vi "SelfieStickControl.vi"(5 "Home Complete":bool, 6 "Arm Position":T23, 7 "Manual Control":dbl, 8 "Inhibit Extend":bool, 9 "Manual Toggle":bool, 10 "Selfie Stick Motor DevRef":T2={"DeviceStatus"={"status"=FALSE, "code"=0, "source"=""}, "Type"=enum."PWM", "PWM"={"PWM Channel"=enum."Invalid", "DeadBand"={"Name"="", "maxPositivePwm"=0, "minPositivePwm"=0, "centerPwm"=0, "maxNegativePwm"=0, "minNegativePwm"=0, "angularRange"=0}}, "CAN"={"Device Number"=0, "SetOutput VI Ref"=variant(enum8{"Percent VBus", "Current", "Speed", "Position", "Voltage"} enum."Percent VBus"), "GetOutput VI Ref"=variant(refnum<k1> refnum), "Enable VI Ref"=variant(dbl 12.0), "Disable VI Ref"=variant(enum8{"Percent VBus", "Speed", "Position", "Slave", "Unchanged / Invalid", "Voltage Compensation", "Current", "Motion Profile"} enum."Percent VBus"), "Data"=variant}, "Invert"=FALSE, "DIO PWM"={"PWM \"Enable\" Channel"=enum."Invalid", "DIOChannel"=enum."Invalid", "PWM Rate"=0.0}}, 11 "RobotConfig":T7={"Motors"={"DriveLeftPrimary"={"CAN Address"=0, "Invert"=FALSE, "InvertSensor"=FALSE, "Unit Conversion Factor"=0.0, "Brake Mode"=enum."Override to Brake", "Reverse Limt Switch Mode"=enum."Normally Closed", "Forward Limt Swith Mode"=enum."Normally Closed", "PWM Channel"=enum."Invalid", "Motor Controller Type"=enum."Talon SRX"}, "DriveLeftSecondary1"={"CAN Address"=0, "Invert"=FALSE, "InvertSensor"=FALSE, "Unit Conversion Factor"=0.0, "Brake Mode"=enum."Override to Brake", "Reverse Limt Switch Mode"=enum."Normally Closed", "Forward Limt Swith Mode"=enum."Normally Closed", "PWM Channel"=enum."Invalid", "Motor Controller Type"=enum."Talon SRX"}, "DriveRightPrimary"={"CAN Address"=0, "Invert"=FALSE, "InvertSensor"=FALSE, "Unit Conversion Factor"=0.0, "Brake Mode"=enum."Override to Brake", "Reverse Limt Switch Mode"=enum."Normally Closed", "Forward Limt Swith Mode"=enum."Normally Closed", "PWM Channel"=enum."Invalid", "Motor Controller Type"=enum."Talon SRX"}, "DriveRightSecondary1"={"CAN Address"=0, "Invert"=FALSE, "InvertSensor"=FALSE, "Unit Conversion Factor"=0.0, "Brake Mode"=enum."Override to Brake", "Reverse Limt Switch Mode"=enum."Normally Closed", "Forward Limt Swith Mode"=enum."Normally Closed", "PWM Channel"=enum."Invalid", "Motor Controller Type"=enum."Talon SRX"}, "RightIntake"={"CAN Address"=8, "Invert"=FALSE, "InvertSensor"=FALSE, "Unit Conversion Factor"=0.0, "Brake Mode"=enum."Override to Brake", "Reverse Limt Switch Mode"=enum."Normally Closed", "Forward Limt Swith Mode"=enum."Normally Closed", "PWM Channel"=enum."Invalid", "Motor Controller Type"=enum."Talon SRX"}, "LeftIntake"={"CAN Address"=7, "Invert"=FALSE, "InvertSensor"=FALSE, "Unit Conversion Factor"=0.0, "Brake Mode"=enum."Override to Brake", "Reverse Limt Switch Mode"=enum."Normally Closed", "Forward Limt Swith Mode"=enum."Normally Closed", "PWM Channel"=enum."Invalid", "Motor Controller Type"=enum."Talon SRX"}, "ArmPivot"={"CAN Address"=5, "Invert"=FALSE, "InvertSensor"=FALSE, "Unit Conversion Factor"=0.0, "Brake Mode"=enum."Override to Brake", "Reverse Limt Switch Mode"=enum."Normally Closed", "Forward Limt Swith Mode"=enum."Normally Closed", "PWM Channel"=enum."Invalid", "Motor Controller Type"=enum."Talon SRX"}, "ArmExtend"={"CAN Address"=6, "Invert"=FALSE, "InvertSensor"=FALSE, "Unit Conversion Factor"=0.0, "Brake Mode"=enum."Override to Brake", "Reverse Limt Switch Mode"=enum."Normally Closed", "Forward Limt Swith Mode"=enum."Normally Closed", "PWM Channel"=enum."Invalid", "Motor Controller Type"=enum."Talon SRX"}, "ArmPivot2"={"CAN Address"=9, "Invert"=FALSE, "InvertSensor"=FALSE, "Unit Conversion Factor"=0.0, "Brake Mode"=enum."Override to Brake", "Reverse Limt Switch Mode"=enum."Normally Closed", "Forward Limt Swith Mode"=enum."Normally Closed", "PWM Channel"=enum."Invalid", "Motor Controller Type"=enum."Talon SRX"}, "Climber"={"CAN Address"=10, "Invert"=FALSE, "InvertSensor"=FALSE, "Unit Conversion Factor"=0.0, "Brake Mode"=enum."Override to Brake", "Reverse Limt Switch Mode"=enum."Disabled", "Forward Limt Swith Mode"=enum."Disabled", "PWM Channel"=enum."Invalid", "Motor Controller Type"=enum."Talon SRX"}, "Selfie Stick"={"CAN Address"=11, "Invert"=FALSE, "InvertSensor"=FALSE, "Unit Conversion Factor"=0.0, "Brake Mode"=enum."Override to Brake", "Reverse Limt Switch Mode"=enum."Disabled", "Forward Limt Swith Mode"=enum."Disabled", "PWM Channel"=enum."Invalid", "Motor Controller Type"=enum."Talon SRX"}}, "Sensors"={"IMU"={"Yaw Axis"=enum."X", "SPI Bus"=enum."SPI MXP", "AHRS Algorithm"=enum."Complementary", "Calibration Time (s)"=3.0, "Calibrate On Open"=FALSE}, "LimitSwitch1"={"DIOChannel"=enum."DIO 0", "Active Low"=FALSE}, "LimitSwitch2"={"DIOChannel"=enum."DIO 1", "Active Low"=FALSE}, "BeamBreak"={"DIOChannel"=enum."DIO 2", "Active Low"=FALSE}, "JeVois"={"Baud Rate"=9600, "Parity"=0, "Data Bits"=8, "Stop Bits"=10, "Termination Char (0xA = '\\n' = LF)"=10, "Enable Termination Char? (T)"=TRUE, "Flow Control"=0, "Timeout Value (ms)"=5000, "Serial Port"=enum."Onboard RS-232"}}, "PID"={"ArmExtend"={"P"=0.0, "I"=0.0, "D"=0.0, "F"=0.0, "IZone"=0.0}, "ArmRotate"={"P"=0.0, "I"=0.0, "D"=0.0, "F"=0.0, "IZone"=0.0}, "Drive"={"P"=0.0, "I"=0.0, "D"=0.0, "F"=0.0, "IZone"=0.0}, "DriveGyro Kp ((in/sec)/deg)"=0.0, "CameraPole"={"P"=0.0, "I"=0.0, "D"=0.0, "F"=0.0, "IZone"=0.0}}, "Solenoids"={"ArmClaw"={"Forward Channel"=enum."Solenoid 0", "Invert"=FALSE, "Reverse Channel"=enum."Solenoid 0"}, "IntakeExtend"={"Forward Channel"=enum."Solenoid 1", "Invert"=FALSE, "Reverse Channel"=enum."Solenoid 0"}, "IntakeOpen"={"Forward Channel"=enum."Solenoid 2", "Invert"=FALSE, "Reverse Channel"=enum."Solenoid 0"}, " Shifter"={"Forward Channel"=enum."Solenoid 3", "Invert"=FALSE, "Reverse Channel"=enum."Solenoid 0"}}, "RobotDimensions "={"Length"=0.0, "Height"=0.0, "HeightOfBumpers"=0.0, "DistanceFromFrameEdgeToPyramid "=0.0, "HeightOfFrameToIntake"=0.0, "EdgeOfFrameToOrigin"=0.0}, "ArmHomePosition"={"Angle (rad)"=0.0, "Radius (in)"=0.0}, "SelfieStickParams"={"Home Height (in)"=0.0, "CruiseVelocity"=0, "MaxAccel"=0, "Low Height (in)"=0.0, "High Height (in)"=0.0, "Mid Height (in)"=0.0}, "Enable Compressor"=TRUE} {"Sensors"."JeVois"."Flow Control" items=["None", "XON/XOFF", "RTS/CTS", "XON/XOFF & RTS/CTS", "DTR/DSR", "XON/XOFF & DTR/DSR"]; "Sensors"."JeVois"."Termination Char (0xA = '\\n' = LF)" format="%.0x"; "Sensors"."JeVois"."Stop Bits" items=["1.0"=10, "1.5"=15, "2.0"=20]; "Sensors"."JeVois"."Parity" items=["None", "Odd", "Even", "Mark", "Space"]}) -> (0 "Selfie Stick State":T1, 3 "Use Arm Camera":bool)   [LabVIEW 2018]
uses:
  Arm/TypeDefs/ArmTargetPosition.ctl
  TypeDefs/ConfigComponents/Config_Robot.ctl
  ArgosLib/Config/ConfigComponents/TypeDefs/Config_Motor.ctl
  <vilib>/Rock Robotics/WPI/ThirdParty/Phoenix-LabVIEW/Motor Controller/Controls/CTRE_Phoenix_MotorControl_NeutralMode.ctl
  <vilib>/Rock Robotics/WPI/ThirdParty/Phoenix-LabVIEW/Motor Controller/Controls/CTRE_Phoenix_MotorControl_LimitSwitchNormal.ctl
  <vilib>/Rock Robotics/SystemInterfaces/DIO/FPGA_DIOPWMChannel.ctl
  ArgosLib/Config/ConfigComponents/TypeDefs/Config_MotorCtrlType.ctl
  ArgosLib/Config/ConfigComponents/TypeDefs/Config_IMU.ctl
  <vilib>/Rock Robotics/SystemInterfaces/spilib/spi_bus.ctl
  ArgosLib/Config/ConfigComponents/TypeDefs/Config_DigitalIO.ctl
  <vilib>/Rock Robotics/SystemInterfaces/DIO/FPGA_DIOChannel.ctl
  ArgosLib/Config/ConfigComponents/TypeDefs/Config_SerialPort.ctl
  <vilib>/Rock Robotics/WPI/SerialPort/WPI_SerialPort.ctl
  ArgosLib/Config/ConfigComponents/TypeDefs/Config_PIDParams.ctl
  ArgosLib/Config/ConfigComponents/TypeDefs/Config_DoubleSolenoid.ctl
  <vilib>/Rock Robotics/WPI/Solenoid/WPI_SolenoidChannel.ctl
  TypeDefs/ConfigComponents/Config_Dimensions.ctl
  TypeDefs/ConfigComponents/Config_ArmHome.ctl
  TypeDefs/ConfigComponents/Config_SelfieStick.ctl
  <vilib>/Rock Robotics/WPI/MotorControl/WPI_MotorControlDeviceRef.ctl
  <vilib>/Rock Robotics/WPI/MotorControl/WPI_MotorControlType.ctl
  <vilib>/Rock Robotics/WPI/PWM/WPI_PWMDeadband.ctl
  TypeDefs/SelfieStickState.ctl
  ArgosLib/Signal Processing/TypeDefs/EdgeDetector_Type.ctl
  <vilib>/Rock Robotics/WPI/ThirdParty/Phoenix-LabVIEW/Motor Controller/Controls/CTRE_Phoenix_MotorControl_ControlMode.ctl
  <vilib>/Rock Robotics/WPI/ThirdParty/Phoenix-LabVIEW/Motor Controller/Get/CTRE_Phoenix_MotorController_GetSelectedSensorData.vi
  ArgosLib/ArgosLib.lvlib
panel:
  out "Position (Raw Sensor Units)":i32
  out "Velocity (Raw Sensor Units per 100 ms)":i32
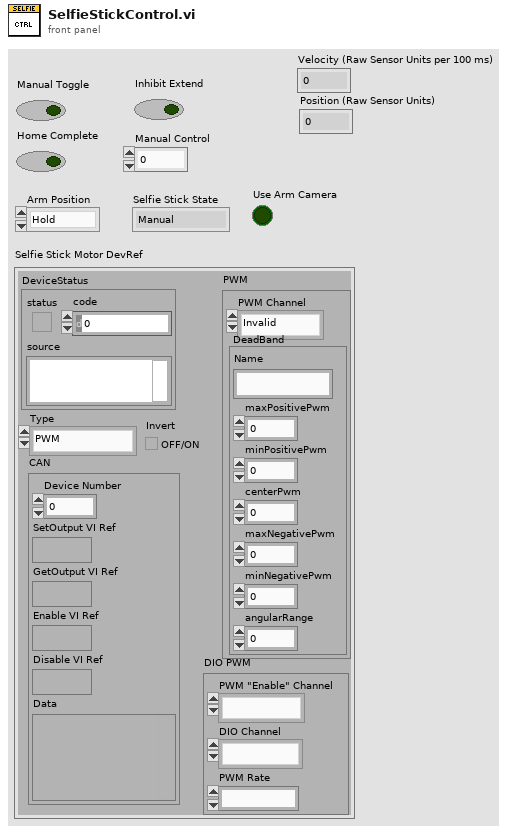
[diagram p1: front panel]
types:
  T1 = typedef "SelfieStickState.ctl" = enum16{"Manual", "Low", "Mid", "High"}
  T2 = typedef "WPI_MotorControlDeviceRef.ctl" = cluster{"DeviceStatus":errorcluster, "Type":T3, "PWM":cluster{"PWM Channel":T4, "DeadBand":T5}, "CAN":cluster{"Device Number":u8, "SetOutput VI Ref":variant, "GetOutput VI Ref":variant, "Enable VI Ref":variant, "Disable VI Ref":variant, "Data":variant}, "Invert":bool, "DIO PWM":cluster{"PWM \"Enable\" Channel":T4, "DIOChannel":T6, "PWM Rate":dbl}}
  T3 = typedef "WPI_MotorControlType.ctl" = enum16{"PWM", "CAN", "DIO PWM"}
  T4 = typedef "FPGA_DIOPWMChannel.ctl" = enum8{"PWM 0", "PWM 1", "PWM 2", "PWM 3", "PWM 4", "PWM 5", "PWM 6", "PWM 7", "PWM 8", "PWM 9", "PWM MXP 0", "PWM MXP 1", "PWM MXP 2", "PWM MXP 3", "PWM MXP 4", "PWM MXP 5", "PWM MXP 6", "PWM MXP 7", "PWM MXP 8", "PWM MXP 9", "Invalid"}
  T5 = typedef "WPI_PWMDeadband.ctl" = cluster{"Name":string, "maxPositivePwm":i32, "minPositivePwm":i32, "centerPwm":i32, "maxNegativePwm":i32, "minNegativePwm":i32, "angularRange":u16}
  T6 = typedef "FPGA_DIOChannel.ctl" = enum8{"DIO 0", "DIO 1", "DIO 2", "DIO 3", "DIO 4", "DIO 5", "DIO 6", "DIO 7", "DIO 8", "DIO 9", "DIO MXP 0", "DIO MXP 1", "DIO MXP 2", "DIO MXP 3", "DIO MXP 4", "DIO MXP 5", "DIO MXP 6", "DIO MXP 7", "DIO MXP 8", "DIO MXP 9", "DIO MXP 10", "DIO MXP 11", "DIO MXP 12", "DIO MXP 13", "DIO MXP 14", "DIO MXP 15", "SPI Port CS1", "SPI Port CS2", "SPI Port CS3", "SPI Port MISO", "SPI Port MOSI", "Invalid"}
  T7 = typedef "Config_Robot.ctl" = cluster{"Motors":cluster{"DriveLeftPrimary":T8, "DriveLeftSecondary1":T8, "DriveRightPrimary":T8, "DriveRightSecondary1":T8, "RightIntake":T8, "LeftIntake":T8, "ArmPivot":T8, "ArmExtend":T8, "ArmPivot2":T8, "Climber":T8, "Selfie Stick":T8}, "Sensors":cluster{"IMU":T12, "LimitSwitch1":T14, "LimitSwitch2":T14, "BeamBreak":T14, "JeVois":T15}, "PID":cluster{"ArmExtend":T17, "ArmRotate":T17, "Drive":T17, "DriveGyro Kp ((in/sec)/deg)":dbl, "CameraPole":T17}, "Solenoids":cluster{"ArmClaw":T18, "IntakeExtend":T18, "IntakeOpen":T18, " Shifter":T18}, "RobotDimensions ":T20, "ArmHomePosition":T21, "SelfieStickParams":T22, "Enable Compressor":bool}
  T8 = typedef "ArgosLib.lvlib/Config_Motor.ctl" = cluster{"CAN Address":u8, "Invert":bool, "InvertSensor":bool, "Unit Conversion Factor":dbl, "Brake Mode":T9, "Reverse Limt Switch Mode":T10, "Forward Limt Swith Mode":T10, "PWM Channel":T4, "Motor Controller Type":T11}
  T9 = typedef "CTRE_Phoenix_MotorControl_NeutralMode.ctl" = enum8{"EEPROMSetting", "Override to Coast", "Override to Brake"}
  T10 = typedef "CTRE_Phoenix_MotorControl_LimitSwitchNormal.ctl" = enum16{"Normally Open", "Normally Closed", "Disabled"}
  T11 = typedef "ArgosLib.lvlib/Config_MotorCtrlType.ctl" = enum16{"Disabled", "Talon SRX", "Talon SR"}
  T12 = typedef "ArgosLib.lvlib/Config_IMU.ctl" = cluster{"Yaw Axis":enum16{"X", "Y", "Z"}, "SPI Bus":T13, "AHRS Algorithm":enum16{"Complementary", "Madgwick"}, "Calibration Time (s)":dbl, "Calibrate On Open":bool}
  T13 = typedef "spi_bus.ctl" = enum16{"SPI On-Board, CS0", "SPI On-Board, CS1", "SPI On-Board, CS2", "SPI On-Board, CS3", "SPI MXP", "Invalid"}
  T14 = typedef "ArgosLib.lvlib/Config_DigitalIO.ctl" = cluster{"DIOChannel":T6, "Active Low":bool}
  T15 = typedef "ArgosLib.lvlib/Config_SerialPort.ctl" = cluster{"Baud Rate":u32, "Parity":u16, "Data Bits":u16, "Stop Bits":u16, "Termination Char (0xA = '\\n' = LF)":u8, "Enable Termination Char? (T)":bool, "Flow Control":u16, "Timeout Value (ms)":u32, "Serial Port":T16}
  T16 = typedef "WPI_SerialPort.ctl" = enum16{"Onboard RS-232", "MXP TTL", "USB 1", "USB 2"}
  T17 = typedef "ArgosLib.lvlib/Config_PIDParams.ctl" = cluster{"P":dbl, "I":dbl, "D":dbl, "F":dbl, "IZone":dbl}
  T18 = typedef "ArgosLib.lvlib/Config_DoubleSolenoid.ctl" = cluster{"Forward Channel":T19, "Invert":bool, "Reverse Channel":T19}
  T19 = typedef "WPI_SolenoidChannel.ctl" = enum8{"Solenoid 0", "Solenoid 1", "Solenoid 2", "Solenoid 3", "Solenoid 4", "Solenoid 5", "Solenoid 6", "Solenoid 7", "Invalid"}
  T20 = typedef "Config_Dimensions.ctl" = cluster{"Length":dbl, "Height":dbl, "HeightOfBumpers":dbl, "DistanceFromFrameEdgeToPyramid ":dbl, "HeightOfFrameToIntake":dbl, "EdgeOfFrameToOrigin":dbl}
  T21 = typedef "Config_ArmHome.ctl" = cluster{"Angle (rad)":dbl, "Radius (in)":dbl}
  T22 = typedef "Config_SelfieStick.ctl" = cluster{"Home Height (in)":dbl, "CruiseVelocity":i32, "MaxAccel":i32, "Low Height (in)":dbl, "High Height (in)":dbl, "Mid Height (in)":dbl}
  T23 = typedef "ArmTargetPosition.ctl" = enum16{"Hold", "Switch", "Scale Low", "Scale High", "Climb", "Back Place"}
  T24 = typedef "ArgosLib.lvlib/EdgeDetector_Type.ctl" = enum16{"RisingEdge", "FallingEdge", "Both"}
  T25 = typedef "CTRE_Phoenix_MotorControl_ControlMode.ctl" = u16
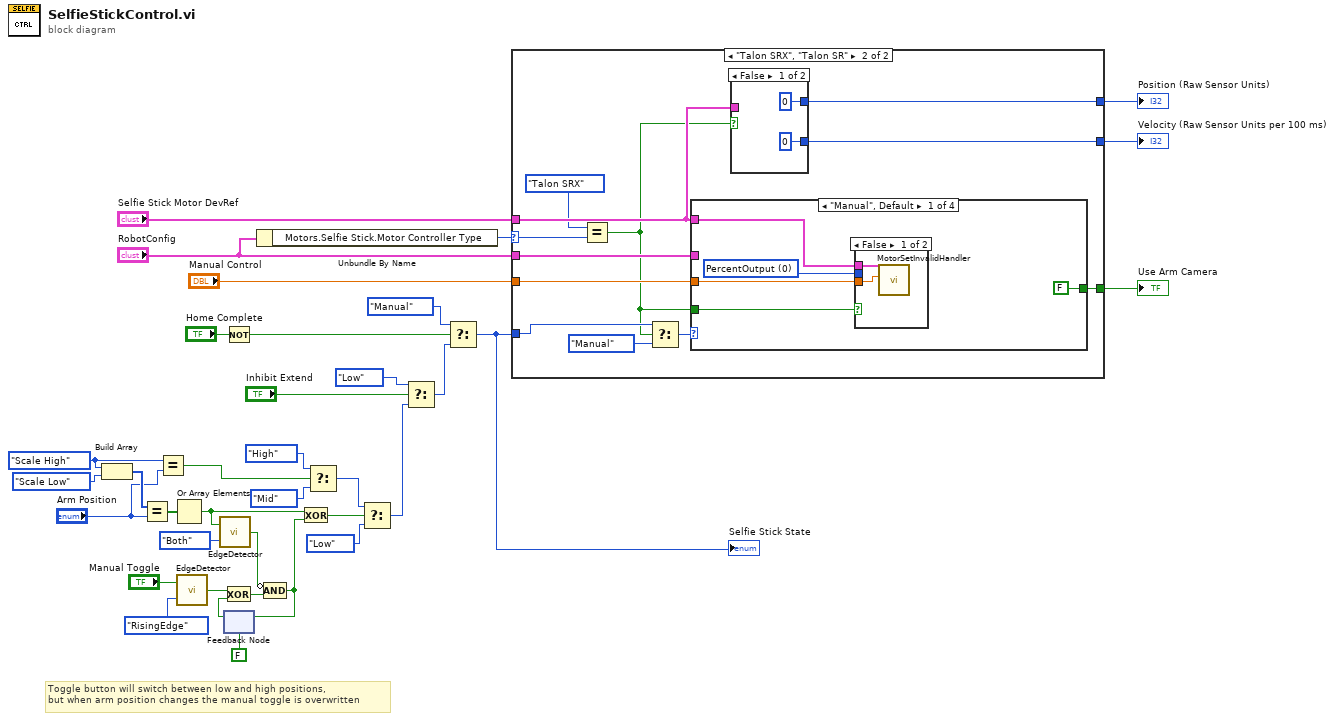
[diagram p0: block diagram]
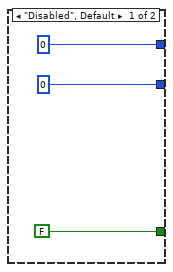
[diagram p2: hidden frame]
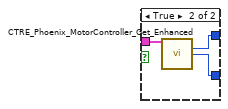
[diagram p3: hidden frame]
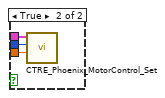
[diagram p4: hidden frame]
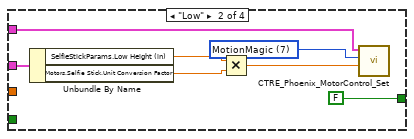
[diagram p5: hidden frame]
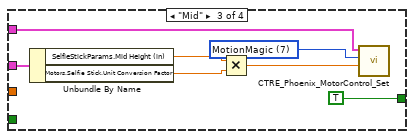
[diagram p6: hidden frame]
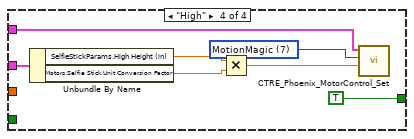
[diagram p7: hidden frame]
diagram:
  w4 = ArmTargetPosition."Scale High" ("Arm Position")
  # "Toggle button will switch between low and high positions,\nbut when arm position changes the manual toggle is overwritten"
  n1 = Build Array(w4, ArmTargetPosition."Scale Low" ("Arm Position")) -> (w29:T23[])
  n2 = Equal?(x=w29, y="Arm Position") -> (x = y?=w28:bool[])
  n3 = Equal?(x=w4, y="Arm Position") -> (x = y?=w3:bool)
  n4 = Or Array Elements(Boolean array=w28) -> (logical OR=w24:bool)
  n5 = call "EdgeDetector.vi"("DetectorType"=EdgeDetector_Type."RisingEdge", "Input"="Manual Toggle") -> ("Edge"=w22:bool)
  n6 = call "EdgeDetector.vi"("DetectorType"=EdgeDetector_Type."Both", "Input"=w24) -> ("Edge"=w18:bool)
  n7 = Not(x="Home Complete") -> (.not. x?=w33:bool)
  n8 = feedback #1(FALSE) -> (w20:bool)
  n9 = Exclusive Or(1:w20, 2:w22) -> (0:w21:bool)
  n10 = Unbundle By Name("RobotConfig") -> ("Motors.Selfie Stick.Motor Controller Type"=w1:T11)
  n11 = Compound Arithmetic op=AND(invert w18, w21) -> (w16:bool)
  n12 = feedback-in #1(w16) -> ()
  n13 = Exclusive Or(1:w16, 2:w24) -> (0:w17:bool)
  n14 = Select(t=SelfieStickState."High" ("Selfie Stick State"), s=w3, f=SelfieStickState."Mid") -> (s? t:f=w8:T1)
  n15 = Select(t=w8, s=w17, f=SelfieStickState."Low" ("Selfie Stick State")) -> (s? t:f=w15:T1)
  n16 = Select(t=SelfieStickState."Low", s="Inhibit Extend", f=w15) -> (s? t:f=w14:T1)
  n17 = Select(t=SelfieStickState."Manual" ("Selfie Stick State"), s=w33, f=w14) -> (s? t:f=w31:T1)
  "Selfie Stick State" <- w31
  n18 = case shown="\"Talon SRX\", \"Talon SR\"" w1 {
    selector: w1 -> [_ w42]
    tunnel: w31 -> [_ w44]
    tunnel: [FALSE w51] -> w13
    tunnel: "Manual Control" -> [_ w50]
    tunnel: "Selfie Stick Motor DevRef" -> [_ w49]
    tunnel: [0 ("Velocity (Raw Sensor Units per 100 ms)") w48] -> w10
    tunnel: [0 ("Position (Raw Sensor Units)") w47] -> w9
    tunnel: "RobotConfig" -> [_ w46]
    frame "Disabled", Default {
    }
    frame "Talon SRX", "Talon SR" {
      n19 = Equal?(x=Config_MotorCtrlType."Talon SRX", y=w42) -> (x = y?=w40:bool)
      n20 = Select(t=w44, s=w40, f=SelfieStickState."Manual") -> (s? t:f=w45:T1)
      n21 = case shown="\"Manual\", Default" w45 {
        tunnel: [FALSE FALSE TRUE TRUE] -> w51
        tunnel: w50 -> [w60 _ _ _]
        tunnel: w49 -> [w58 w68 w75 w82]
        tunnel: w46 -> [_ w72 w79 w86]
        tunnel: w40 -> [w57 _ _ _]
        frame "Manual", Default {
          w59 = T25 0 items=["PercentOutput"=0, "Position"=1, "Velocity"=2, "Current"=3, "Follower"=5, "MotionProfile"=6, "MotionMagic"=7, "MotionMagicArc"=8, "MotionProfileArc"=10, "Disabled"=15] ("Control Mode")
          n22 = case shown="False" w57 {
            tunnel: w60 -> [w62 w66]
            tunnel: w59 -> [_ w65]
            tunnel: w58 -> [w63 w64]
            frame False {
              n23 = call "MotorSetInvalidHandler.vi"("Output"=w62, "MotorControlDevRef"=w63) -> ()  [unwired: 7 in, 3 out]
            }
            frame True {
              n24 = call <vilib>:"CTRE_Phoenix_MotorControl_Set.vi"("Output"=w66, "Control Mode"=w65, "PhoenixMotorControlDevRef"=w64) -> ()  [unwired: 7 in, 2 out]
            }
          }
        }
        frame "Low" {
          w67 = T25 7 items=["PercentOutput"=0, "Position"=1, "Velocity"=2, "Current"=3, "Follower"=5, "MotionProfile"=6, "MotionMagic"=7, "MotionMagicArc"=8, "MotionProfileArc"=10, "Disabled"=15] ("Control Mode")
          n25 = Unbundle By Name(w72) -> ("SelfieStickParams.Low Height (in)"=w71:dbl, "Motors.Selfie Stick.Unit Conversion Factor"=w70:dbl)
          n26 = Multiply(x=w71, y=w70) -> (x*y=w69:dbl)
          n27 = call <vilib>:"CTRE_Phoenix_MotorControl_Set.vi"("Output"=w69, "Control Mode"=w67, "PhoenixMotorControlDevRef"=w68) -> ()  [unwired: 7 in, 2 out]
        }
        frame "Mid" {
          w74 = T25 7 items=["PercentOutput"=0, "Position"=1, "Velocity"=2, "Current"=3, "Follower"=5, "MotionProfile"=6, "MotionMagic"=7, "MotionMagicArc"=8, "MotionProfileArc"=10, "Disabled"=15] ("Control Mode")
          n28 = Unbundle By Name(w79) -> ("SelfieStickParams.Mid Height (in)"=w78:dbl, "Motors.Selfie Stick.Unit Conversion Factor"=w77:dbl)
          n29 = Multiply(x=w78, y=w77) -> (x*y=w76:dbl)
          n30 = call <vilib>:"CTRE_Phoenix_MotorControl_Set.vi"("Output"=w76, "Control Mode"=w74, "PhoenixMotorControlDevRef"=w75) -> ()  [unwired: 7 in, 2 out]
        }
        frame "High" {
          w81 = T25 7 items=["PercentOutput"=0, "Position"=1, "Velocity"=2, "Current"=3, "Follower"=5, "MotionProfile"=6, "MotionMagic"=7, "MotionMagicArc"=8, "MotionProfileArc"=10, "Disabled"=15] ("Control Mode")
          n31 = Unbundle By Name(w86) -> ("SelfieStickParams.High Height (in)"=w85:dbl, "Motors.Selfie Stick.Unit Conversion Factor"=w84:dbl)
          n32 = Multiply(x=w85, y=w84) -> (x*y=w83:dbl)
          n33 = call <vilib>:"CTRE_Phoenix_MotorControl_Set.vi"("Output"=w83, "Control Mode"=w81, "PhoenixMotorControlDevRef"=w82) -> ()  [unwired: 7 in, 2 out]
        }
      }
      n34 = case shown="False" w40 {
        tunnel: w49 -> [_ w56]
        tunnel: [0 ("Velocity (Raw Sensor Units per 100 ms)") w55] -> w48
        tunnel: [0 ("Position (Raw Sensor Units)") w54] -> w47
        frame False {
        }
        frame True {
          n35 = call-poly <vilib>:"CTRE_Phoenix_MotorController_Get_Enhanced.vi"("PhoenixMotorControlDevRef"=w56) -> ("Position (Raw Sensor Units)"=w54:i32, "Velocity (Raw Sensor Units per 100 ms)"=w55:i32)  [unwired: 11 in, 2 out]
        }
      }
    }
  }
  "Use Arm Camera" <- w13
  "Velocity (Raw Sensor Units per 100 ms)" <- w10
  "Position (Raw Sensor Units)" <- w9
